vi "4Pi Dual DM - Text Modes.vi"(7 "Mirror Modes In":T1) -> (4 "Modes 01":string, 15 "Modes 02":string)   [LabVIEW 2020]
uses:
  4Pi Dual DM - Controls/4Pi Dual DM - Mirror Modes DUAL.ctl
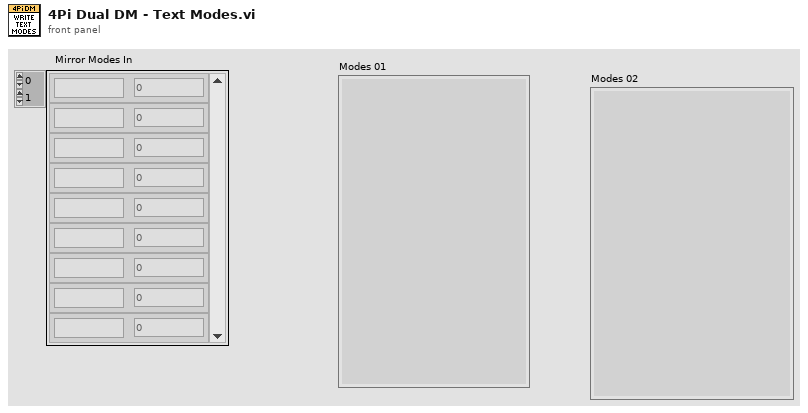
[diagram p1: front panel]
types:
  T1 = typedef "4Pi Dual DM - Mirror Modes DUAL.ctl" = cluster{"Mode":string, "Amplitude":dbl}[][]
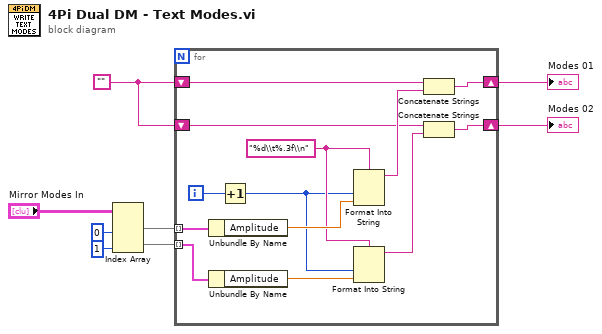
[diagram p0: block diagram]
diagram:
  w4 = ""
  n1 = Index Array(array="Mirror Modes In", index (col) #1=0 ("disabled index (col)"), index (col) #2=1 ("index (col)")) -> (element #1=w6:cluster{"Mode":string, "Amplitude":dbl}[], element #2=w5:cluster{"Mode":string, "Amplitude":dbl}[])  [unwired: 2 in]
  n2 = for {
    tunnel: w6 -> [w21] mode=indexing
    tunnel: w5 -> [w20] mode=indexing
    shift-right: [w9] -> w1
    shift-left: w4 -> [w14]
    shift-right: [w10] -> w2
    shift-left: w4 -> [w12]
    i -> [w19]
    w17 = "%d\\t%.3f\\n" ("format string")
    n3 = Unbundle By Name(w21) -> ("Amplitude"=w18:dbl)
    n4 = Unbundle By Name(w20) -> ("Amplitude"=w16:dbl)
    n5 = Increment(x=w19) -> (x+1=w15:i32)
    n6 = Format Into String(format string=w17, w15, w18) -> (resulting string=w13:string)  [unwired: 2 in, 1 out]
    n7 = Format Into String(format string=w17, w15, w16) -> (resulting string=w11:string)  [unwired: 2 in, 1 out]
    n8 = Concatenate Strings(w14, w13) -> (w9:string)
    n9 = Concatenate Strings(w12, w11) -> (w10:string)
  }
  "Modes 01" <- w1
  "Modes 02" <- w2
